vi "Ev bp.vi"(8 "error in (no error)":errorcluster, 11 "IDE simple in":refnum<class "Main Panel.lvclass">) -> (0 "error out":errorcluster, 3 "IDE simple out":refnum<class "Main Panel.lvclass">)   [LabVIEW 2018, in "Main Panel.lvlib" / "Main Panel.lvclass"]
uses:
  Main Panel.lvclass
  Main Panel.lvclass/Main Panel.ctl
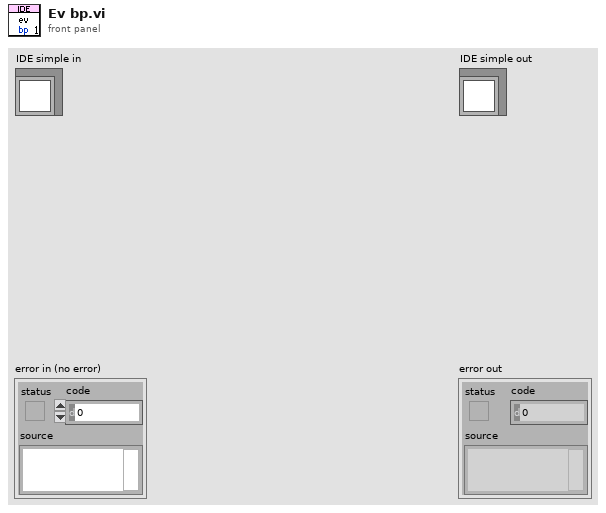
[diagram p1: front panel]
types:
  T1 = typedef "Data Parser.lvclass/frame bp data.ctl" = cluster{"x":string, "y":string}
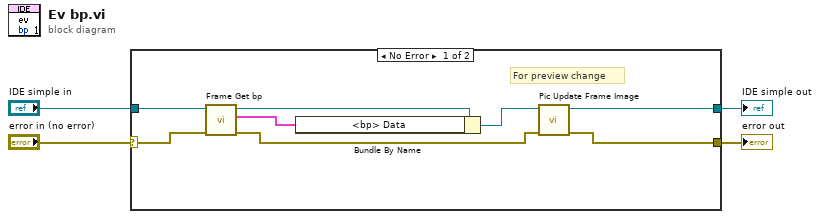
[diagram p0: block diagram]
diagram:
  n1 = case shown="No Error" "error in (no error)" {
    selector: "error in (no error)" -> [w11 w14]
    tunnel: [w5 w14] -> w3
    tunnel: [w6 w13] -> w1
    tunnel: "IDE simple in" -> [w12 w13]
    frame No Error {
      # "For preview change"
      n2 = call "Frame Get bp.vi"("error in (no error)"=w11, "IDE simple in"=w12) -> ("error out"=w7:errorcluster, "<bp> Data"=w9:T1, "IDE simple out"=w10:refnum<class "Main Panel.lvclass">)  [unwired: 7 in]
      n3 = Bundle By Name(cluster=w10, "<bp> Data"=w9) -> (w8:refnum<class "Main Panel.lvclass">)
      n4 = call "Pic Update Frame Image.vi"("error in (no error)"=w7, "LF2R IDE in"=w8) -> ("error out"=w5:errorcluster, "LF2R IDE out"=w6:refnum<class "Main Panel.lvclass">)  [unwired: 8 in]
    }
    frame Error {
    }
  }
  "error out" <- w3
  "IDE simple out" <- w1
